vi "RTS Volt Freq CMD Update.vi"(8 "Error In":errorcluster, 9 "Data String":string, 10 "Station Number":string, 11 "Device Connections In":T1 {"MX5"."Channel Number (1)" min=1 max=60 step=1; "MX5"."FIFO Number (0)" min=-1 max=2 step=1; "MX4"."Channel Number (1)" min=1 max=60 step=1; "MX4"."FIFO Number (0)" min=-1 max=2 step=1; "MX3"."Channel Number (1)" min=1 max=60 step=1; "MX3"."FIFO Number (0)" min=-1 max=2 step=1; "MX2"."Channel Number (1)" min=1 max=60 step=1; "MX2"."FIFO Number (0)" min=-1 max=2 step=1; "MX1"."Channel Number (1)" min=1 max=60 step=1; "MX1"."FIFO Number (0)" min=-1 max=2 step=1}) -> (0 "Error Out":errorcluster, 3 "Device Connections Out":T1={"Wago ModBus Connection"=refnum, "APLUS 1 Modbus Connection"=refnum, "APLUS 2 Modbus Connection"=refnum, "APLUS 3 Modbus Connection"=refnum, "APLUS 4 Modbus Connection"=refnum, "APLUS 5 Modbus Connection"=refnum, "APLUS 6 Modbus Connection"=refnum, "APLUS 7 Modbus Connection"=refnum, "APLUS 8 Modbus Connection"=refnum, "MX 1 VISA Connection"="", "MX 2 VISA Connection"="", "MX 3 VISA Connection"="", "MX 4 VISA Connection"="", "MX 5 VISA Connection"="", "MX1"={"Base Time"=0, "Session Number"=0, "Last Data Number"={"High"=-1, "Low"=4294967295}, "Channel List"=[], "FIFO Number (0)"=0, "Channel Number (1)"=1, "Select FIFO or Channel (F:Channel)"=FALSE, "MX100 Data"={"Measurement Values out"=[], "Date/Time"=""}}, "MX2"={"Base Time"=0, "Session Number"=0, "Last Data Number"={"High"=-1, "Low"=4294967295}, "Channel List"=[], "FIFO Number (0)"=0, "Channel Number (1)"=1, "Select FIFO or Channel (F:Channel)"=FALSE, "MX100 Data"={"Measurement Values out"=[], "Date/Time"=""}}, "MX3"={"Base Time"=0, "Session Number"=0, "Last Data Number"={"High"=-1, "Low"=4294967295}, "Channel List"=[], "FIFO Number (0)"=0, "Channel Number (1)"=1, "Select FIFO or Channel (F:Channel)"=FALSE, "MX100 Data"={"Measurement Values out"=[], "Date/Time"=""}}, "MX4"={"Base Time"=0, "Session Number"=0, "Last Data Number"={"High"=-1, "Low"=4294967295}, "Channel List"=[], "FIFO Number (0)"=0, "Channel Number (1)"=1, "Select FIFO or Channel (F:Channel)"=FALSE, "MX100 Data"={"Measurement Values out"=[], "Date/Time"=""}}, "MX5"={"Base Time"=0, "Session Number"=0, "Last Data Number"={"High"=-1, "Low"=4294967295}, "Channel List"=[], "FIFO Number (0)"=0, "Channel Number (1)"=1, "Select FIFO or Channel (F:Channel)"=FALSE, "MX100 Data"={"Measurement Values out"=[], "Date/Time"=""}}} {"MX5"."Channel Number (1)" min=1 max=60 step=1; "MX5"."FIFO Number (0)" min=-1 max=2 step=1; "MX4"."Channel Number (1)" min=1 max=60 step=1; "MX4"."FIFO Number (0)" min=-1 max=2 step=1; "MX3"."Channel Number (1)" min=1 max=60 step=1; "MX3"."FIFO Number (0)" min=-1 max=2 step=1; "MX2"."Channel Number (1)" min=1 max=60 step=1; "MX2"."FIFO Number (0)" min=-1 max=2 step=1; "MX1"."Channel Number (1)" min=1 max=60 step=1; "MX1"."FIFO Number (0)" min=-1 max=2 step=1})   [LabVIEW 2016]
uses:
  Type Definitions/RTS Modbus Connections.ctl
  <vilib>/NI/Modbus Library/API/Master/Modbus Master.lvclass
  Drivers/Yokogawa MX100/Type Definitions/MX100 Initialization.ctl
  Drivers/Yokogawa MX100/Type Definitions/MX100 Data.ctl
panel:
  # "Volt-0.00,Freq-0,RstWh-1"
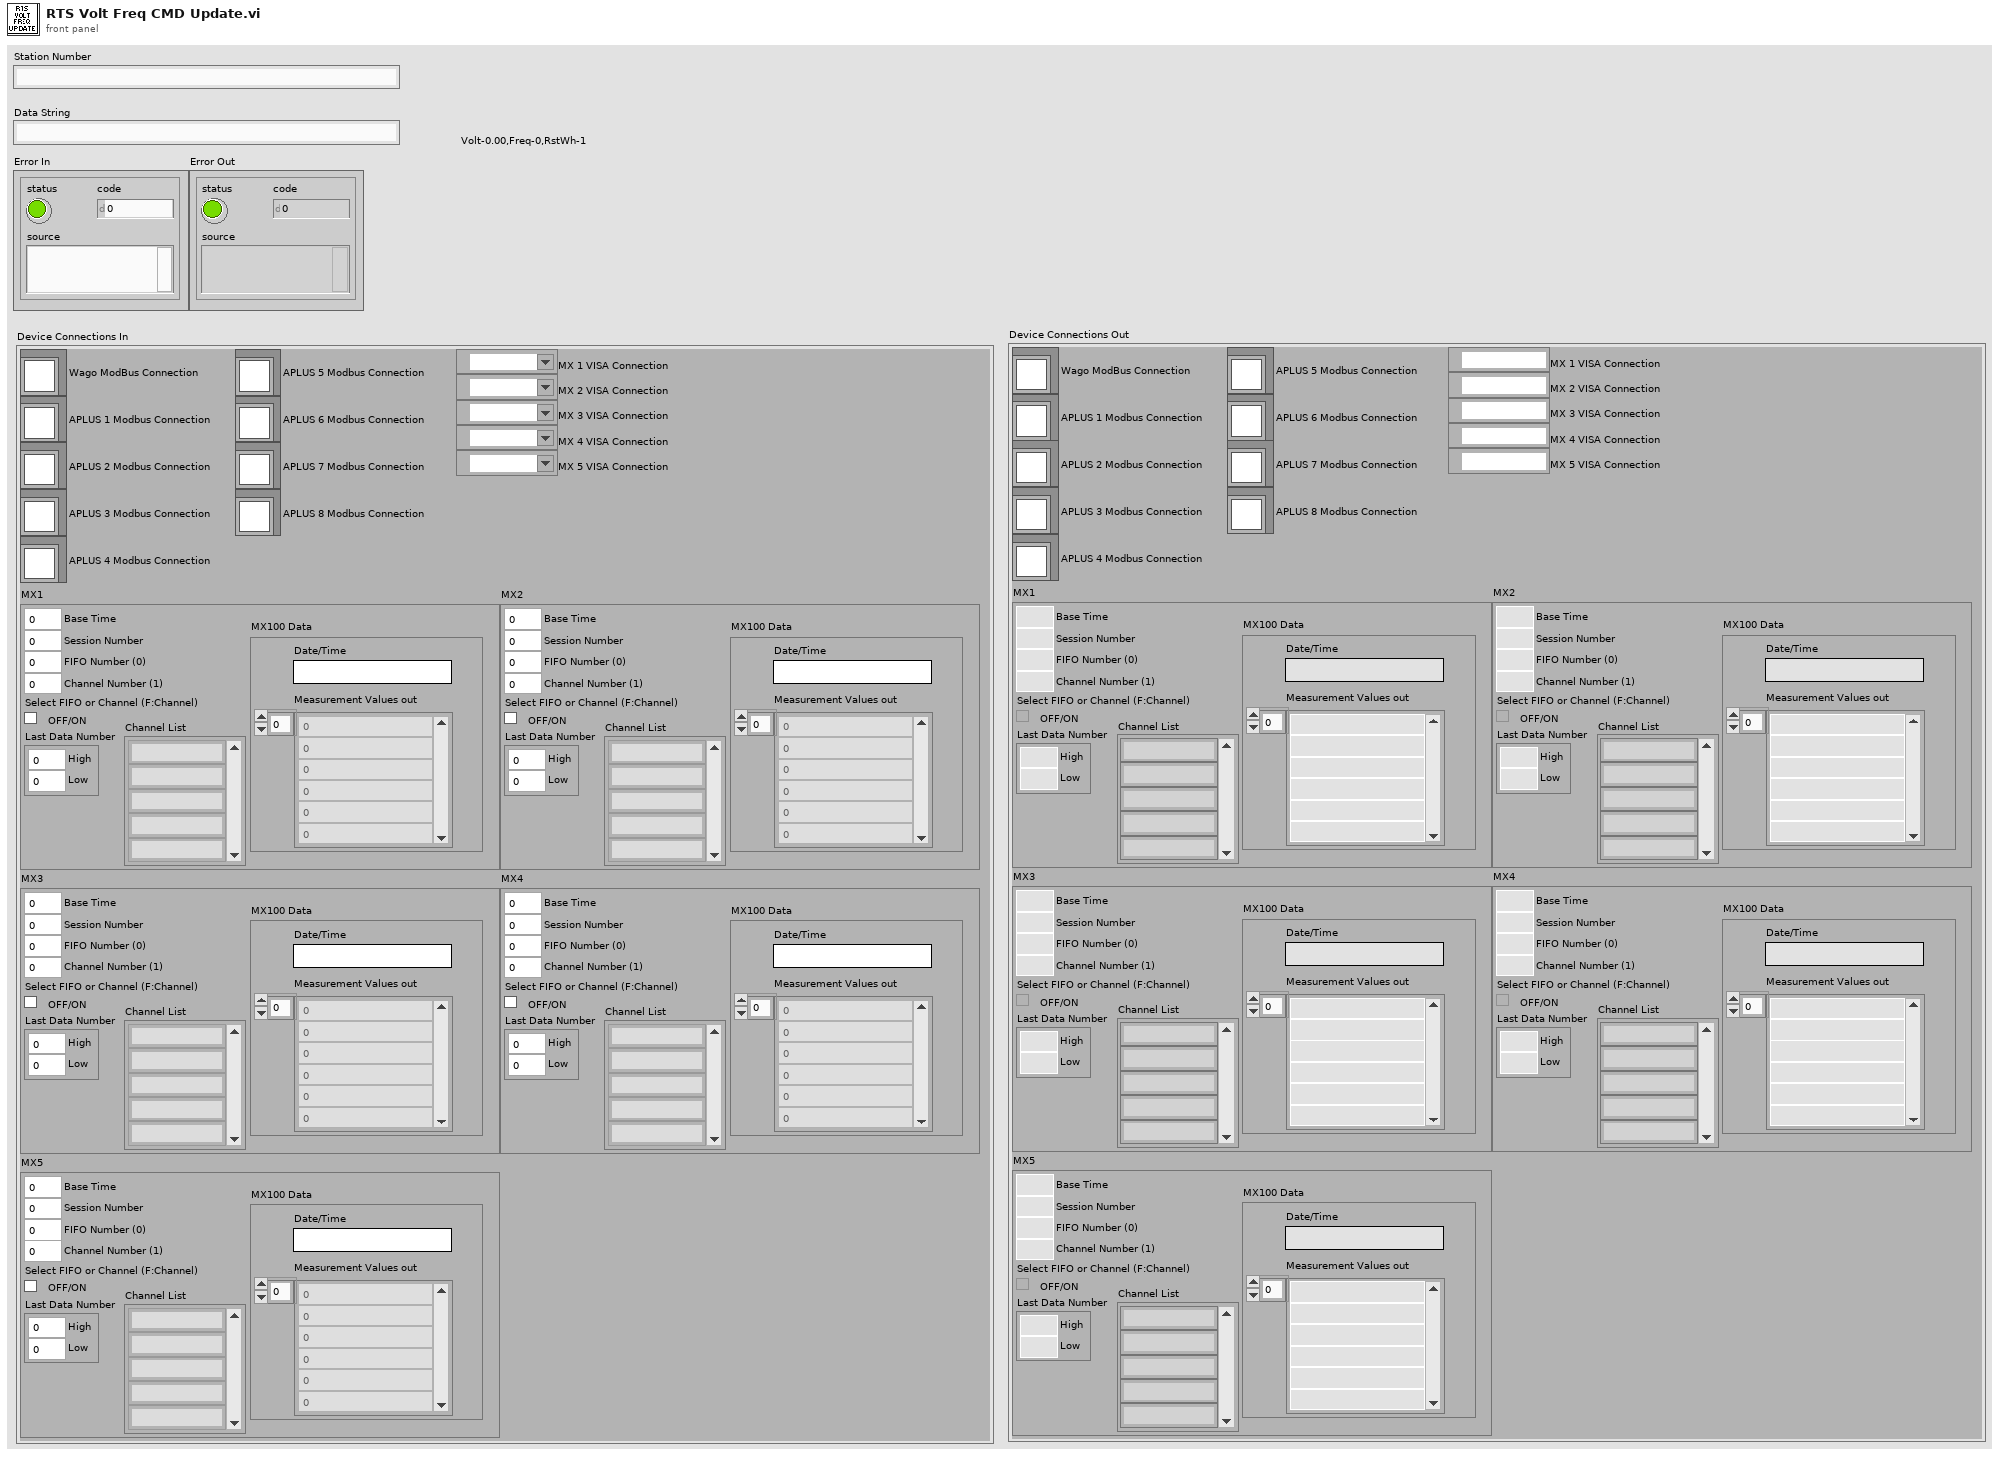
[diagram p1: front panel]
types:
  T1 = typedef "RTS Modbus Connections.ctl" = cluster{"Wago ModBus Connection":refnum<class "Modbus Master.lvclass">, "APLUS 1 Modbus Connection":refnum<class "Modbus Master.lvclass">, "APLUS 2 Modbus Connection":refnum<class "Modbus Master.lvclass">, "APLUS 3 Modbus Connection":refnum<class "Modbus Master.lvclass">, "APLUS 4 Modbus Connection":refnum<class "Modbus Master.lvclass">, "APLUS 5 Modbus Connection":refnum<class "Modbus Master.lvclass">, "APLUS 6 Modbus Connection":refnum<class "Modbus Master.lvclass">, "APLUS 7 Modbus Connection":refnum<class "Modbus Master.lvclass">, "APLUS 8 Modbus Connection":refnum<class "Modbus Master.lvclass">, "MX 1 VISA Connection":refnum<visa-resource-name>, "MX 2 VISA Connection":refnum<visa-resource-name>, "MX 3 VISA Connection":refnum<visa-resource-name>, "MX 4 VISA Connection":refnum<visa-resource-name>, "MX 5 VISA Connection":refnum<visa-resource-name>, "MX1":T2, "MX2":T2, "MX3":T2, "MX4":T2, "MX5":T2}
  T2 = typedef "MX100 Initialization.ctl" = cluster{"Base Time":i32, "Session Number":i32, "Last Data Number":cluster{"High":i32, "Low":u32}, "Channel List":string[], "FIFO Number (0)":i32, "Channel Number (1)":i32, "Select FIFO or Channel (F:Channel)":bool, "MX100 Data":T3}
  T3 = typedef "MX100 Data.ctl" = cluster{"Measurement Values out":dbl[], "Date/Time":string}
  T4 = typedef "RTS Frequency Selector.ctl" = u16
  T5 = typedef "RTS Reset Watt Hours.ctl" = enum16{"", "Reset Watt Hours"}
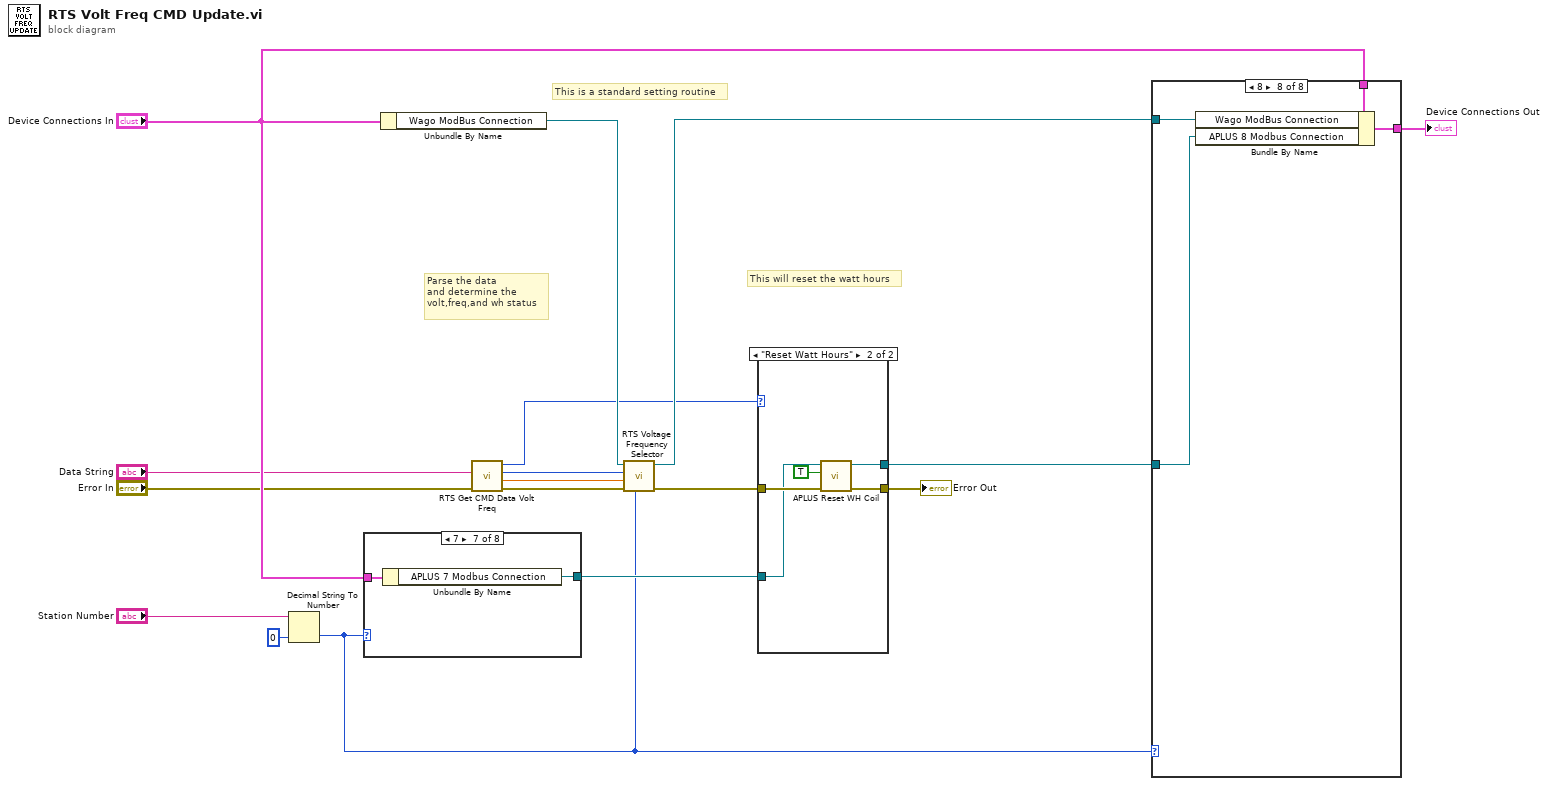
[diagram p0: block diagram]
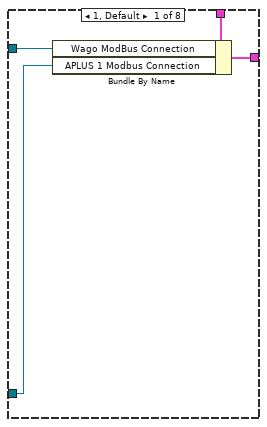
[diagram p2: hidden frame]
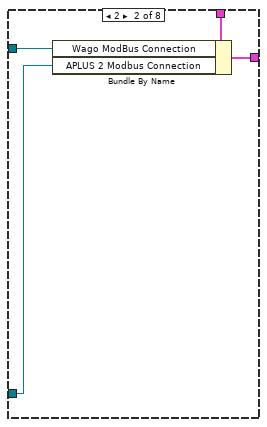
[diagram p3: hidden frame]
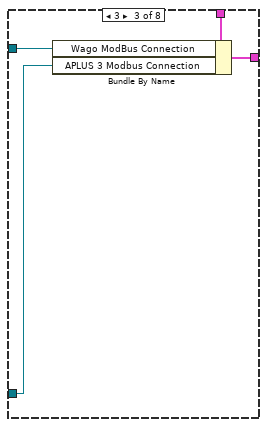
[diagram p4: hidden frame]
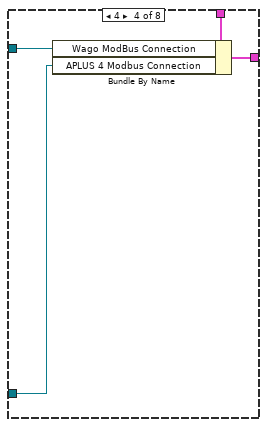
[diagram p5: hidden frame]
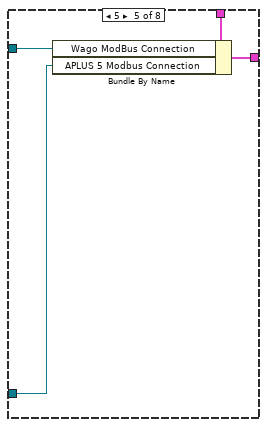
[diagram p6: hidden frame]
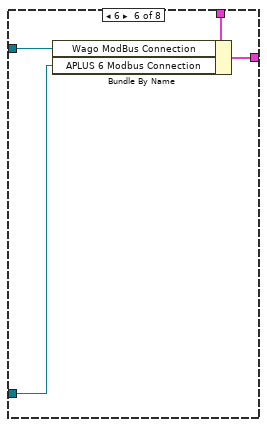
[diagram p7: hidden frame]
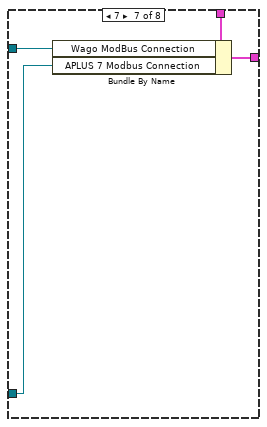
[diagram p8: hidden frame]
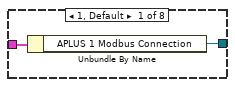
[diagram p9: hidden frame]
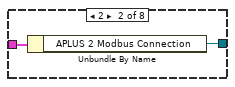
[diagram p10: hidden frame]
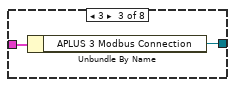
[diagram p11: hidden frame]
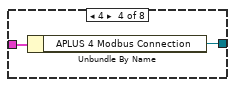
[diagram p12: hidden frame]
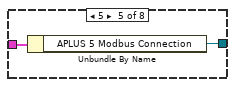
[diagram p13: hidden frame]
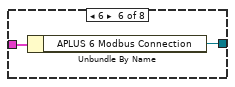
[diagram p14: hidden frame]
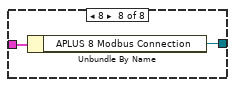
[diagram p15: hidden frame]
diagram:
  # "This will reset the watt hours"
  # "This is a standard setting routine"
  # "Parse the data\nand determine the \nvolt,freq,and wh status"
  n1 = Decimal String To Number(string="Station Number", default (0L)=u16 0 ("default (0 I32)")) -> (number=w2:u16)  [unwired: 1 in, 1 out]
  n2 = case shown="7" w2 {
    tunnel: "Device Connections In" -> [w19 w21 w23 w25 w27 w29 w31 w33]
    tunnel: [w18 w20 w22 w24 w26 w28 w30 w32] -> w11
    frame 1, Default {
      n3 = Unbundle By Name(w19) -> ("APLUS 1 Modbus Connection"=w18:refnum<class "Modbus Master.lvclass">)
    }
    frame 2 {
      n4 = Unbundle By Name(w21) -> ("APLUS 2 Modbus Connection"=w20:refnum<class "Modbus Master.lvclass">)
    }
    frame 3 {
      n5 = Unbundle By Name(w23) -> ("APLUS 3 Modbus Connection"=w22:refnum<class "Modbus Master.lvclass">)
    }
    frame 4 {
      n6 = Unbundle By Name(w25) -> ("APLUS 4 Modbus Connection"=w24:refnum<class "Modbus Master.lvclass">)
    }
    frame 5 {
      n7 = Unbundle By Name(w27) -> ("APLUS 5 Modbus Connection"=w26:refnum<class "Modbus Master.lvclass">)
    }
    frame 6 {
      n8 = Unbundle By Name(w29) -> ("APLUS 6 Modbus Connection"=w28:refnum<class "Modbus Master.lvclass">)
    }
    frame 7 {
      n9 = Unbundle By Name(w31) -> ("APLUS 7 Modbus Connection"=w30:refnum<class "Modbus Master.lvclass">)
    }
    frame 8 {
      n10 = Unbundle By Name(w33) -> ("APLUS 8 Modbus Connection"=w32:refnum<class "Modbus Master.lvclass">)
    }
  }
  n11 = Unbundle By Name("Device Connections In") -> ("Wago ModBus Connection"=w15:refnum<class "Modbus Master.lvclass">)
  n12 = call "RTS Get CMD Data Volt Freq.vi"("Error In"="Error In", "Data String"="Data String") -> ("Error Out"=w5:errorcluster, "Voltage"=w10:dbl, "Frequency"=w9:T4, "Wh Reset 2"=w7:T5)  [unwired: 6 in]
  n13 = call "RTS Voltage Frequency Selector.vi"("Frequency"=w9, "Station Number"=w2, "Voltage"=w10, "error in (no error)"=w5, "Modbus Master in"=w15) -> ("error out"=w14:errorcluster, "Modbus master out"=w16:refnum<class "Modbus Master.lvclass">)  [unwired: 5 in]
  n14 = case shown="\"Reset Watt Hours\"" w7 {
    tunnel: w14 -> [w35 w38]
    tunnel: [w35 w39] -> w3
    tunnel: w11 -> [w34 w37]
    tunnel: [w34 w36] -> w1
    frame "", Default {
    }
    frame "Reset Watt Hours" {
      n15 = call "APLUS Reset WH Coil.vi"("Error In"=w38, "Reset WattHours"=TRUE, "Modbus Master in"=w37) -> ("Error Out"=w39:errorcluster, "Modbus Master out"=w36:refnum<class "Modbus Master.lvclass">)  [unwired: 7 in]
    }
  }
  "Error Out" <- w3
  n16 = case shown="8" w2 {
    tunnel: w16 -> [w44 w45 w49 w54 w58 w62 w66 w70]
    tunnel: [w43 w47 w51 w55 w59 w63 w67 w71] -> w13
    tunnel: "Device Connections In" -> [w42 w48 w52 w56 w60 w64 w68 w72]
    tunnel: w1 -> [w41 w46 w50 w53 w57 w61 w65 w69]
    frame 1, Default {
      n17 = Bundle By Name(cluster=w42, "Wago ModBus Connection"=w44, "APLUS 1 Modbus Connection"=w41) -> (w43:T1)
    }
    frame 2 {
      n18 = Bundle By Name(cluster=w48, "Wago ModBus Connection"=w45, "APLUS 2 Modbus Connection"=w46) -> (w47:T1)
    }
    frame 3 {
      n19 = Bundle By Name(cluster=w52, "Wago ModBus Connection"=w49, "APLUS 3 Modbus Connection"=w50) -> (w51:T1)
    }
    frame 4 {
      n20 = Bundle By Name(cluster=w56, "Wago ModBus Connection"=w54, "APLUS 4 Modbus Connection"=w53) -> (w55:T1)
    }
    frame 5 {
      n21 = Bundle By Name(cluster=w60, "Wago ModBus Connection"=w58, "APLUS 5 Modbus Connection"=w57) -> (w59:T1)
    }
    frame 6 {
      n22 = Bundle By Name(cluster=w64, "Wago ModBus Connection"=w62, "APLUS 6 Modbus Connection"=w61) -> (w63:T1)
    }
    frame 7 {
      n23 = Bundle By Name(cluster=w68, "Wago ModBus Connection"=w66, "APLUS 7 Modbus Connection"=w65) -> (w67:T1)
    }
    frame 8 {
      n24 = Bundle By Name(cluster=w72, "Wago ModBus Connection"=w70, "APLUS 8 Modbus Connection"=w69) -> (w71:T1)
    }
  }
  "Device Connections Out" <- w13
